vi "saveToDisk.vi"(7 "File Path":path, 8 "error in (no error)":errorcluster, 11 "Flattened Image":T1) -> (0 "error out":errorcluster)   [LabVIEW 2018, in "Image_Diff.lvlib"]
uses:
  Image_Diff.lvlib
  <vilib>/picture/picture.llb/imagedata.ctl
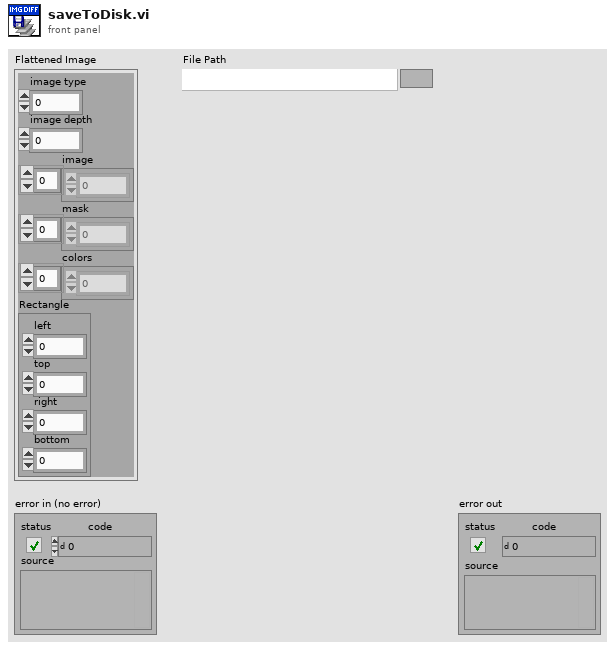
[diagram p1: front panel]
types:
  T1 = typedef "imagedata.ctl" = cluster{"image type":i32, "image depth":i32, "image":u8[], "mask":u8[], "colors":u32[], "Rectangle":cluster{"left":i16, "top":i16, "right":i16, "bottom":i16}}
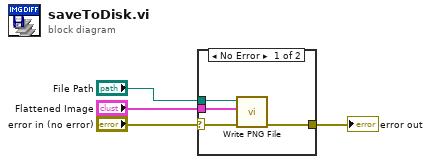
[diagram p0: block diagram]
diagram:
  n1 = case shown="No Error" "error in (no error)" {
    selector: "error in (no error)" -> [w5 w9]
    tunnel: "Flattened Image" -> [w8 _]
    tunnel: "File Path" -> [w7 _]
    tunnel: [w6 w9] -> w2
    frame No Error {
      n2 = call <vilib>:"Write PNG File.vi"("error in (no error)"=w5, "image data"=w8, "path to PNG file"=w7) -> ("error out"=w6:errorcluster)  [unwired: 7 in, 1 out]
    }
    frame Error {
    }
  }
  "error out" <- w2
